vi "Log Data DBL.vi"(7 "Identifier":string, 8 "error in":errorcluster, 9 "Time Stamp":timestamp format="%<%x %.3X>T", 10 "Data":dbl, 11 "IDataLogger in":refnum<class "ILog Data.lvclass">) -> (0 "error out":errorcluster, 3 "IDataLogger out":refnum<class "ILog Data.lvclass">)   [LabVIEW 2024, in "ILog Data.lvclass"]
uses:
  ILog Data.lvclass
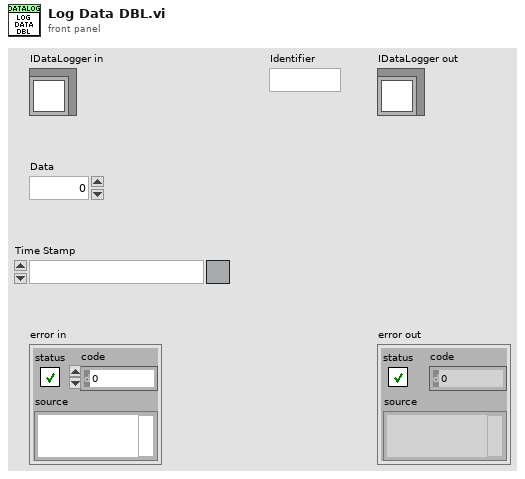
[diagram p1: front panel]
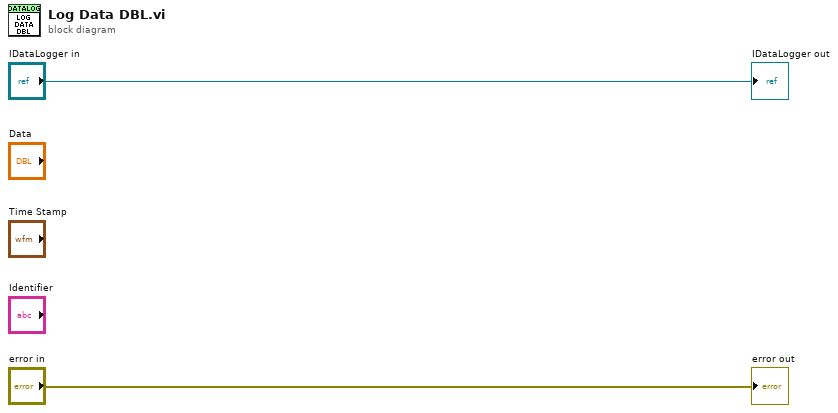
[diagram p0: block diagram]
diagram:
  "error out" <- "error in"
  "IDataLogger out" <- "IDataLogger in"
